vi "Prefix String.vi"(8 "error in (no error)":errorcluster, 10 "Input String":string, 11 "JSON Serializer in":refnum<class "JSON Serializer.lvclass">) -> (0 "error out":errorcluster, 2 "Output String":string, 3 "JSON Serializer out":refnum<class "JSON Serializer.lvclass">)   [LabVIEW 2013, in "JKI JSON Serialization.lvlib" / "JSON Serializer.lvclass"]
uses:
  JSON Serializer.lvclass
  JSON Serializer.lvclass/JSON Serializer.ctl
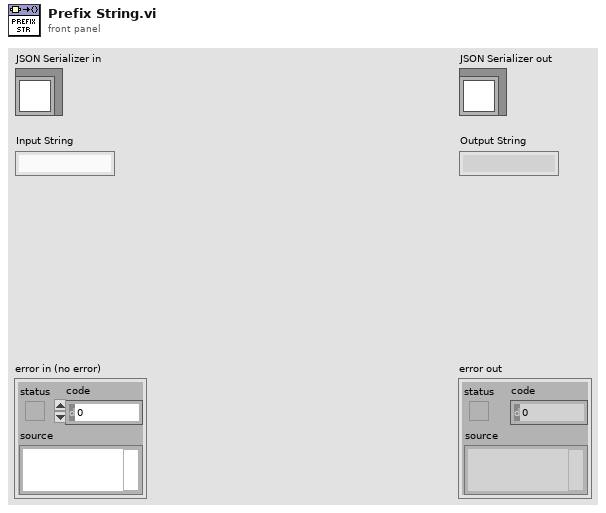
[diagram p1: front panel]
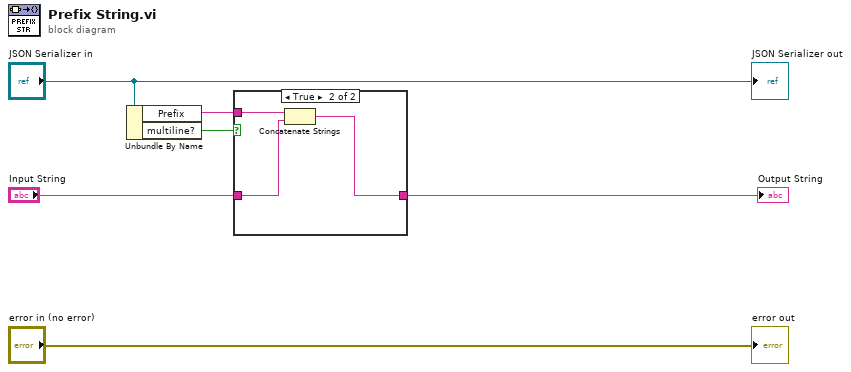
[diagram p0: block diagram]
diagram:
  n1 = Unbundle By Name("JSON Serializer in") -> ("Prefix"=w4:string, "multiline?"=w1:bool)
  n2 = case shown="True" w1 {
    tunnel: w4 -> [_ w10]
    tunnel: "Input String" -> [w7 w9]
    tunnel: [w7 w8] -> w2
    frame False {
    }
    frame True {
      n3 = Concatenate Strings(w10, w9) -> (w8:string)
    }
  }
  "Output String" <- w2
  "error out" <- "error in (no error)"
  "JSON Serializer out" <- "JSON Serializer in"
